vi "Figura_SubVi.vi"(10 "string":string, 11 "Path":path) -> (3 "picture":picture)   [LabVIEW 2014]
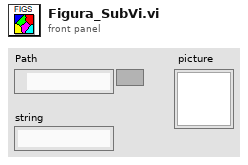
[diagram p1: front panel]
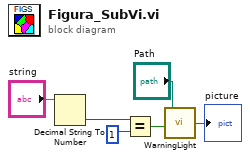
[diagram p0: block diagram]
diagram:
  n1 = Decimal String To Number(string="string") -> (number=w4:i32)  [unwired: 2 in, 1 out]
  n2 = Equal?(x=w4, y=1) -> (x = y?=w3:bool)
  n3 = call "WarningLight.vi"("Boolean"=w3, "Path"="Path") -> ("new picture"=→"picture":picture)
